vi "SentinelController v35 good v11.vi"() -> ()   [LabVIEW 2011] (continued)
                                n1227 = local read "GPIB Bus 0 traffic"() -> (w1138:string)
                                n1228 = Concatenate Strings(w1138, "\r\n", "Bus 0 waiting on SPOLL" ("string")) -> (w1135:string)
                                n1229 = local write "GPIB Bus 0 traffic"(w1135) -> ()
                                }
                                frame #1 {
                                n1230 = local read "VISA bus 0 resource name out hid"() -> (w1139:refnum<visa-resource-name>)
                                n1231 = local read "VISA bus 0 error out hid"() -> (w1140:errorcluster)
                                n1232 = VISA Discard Events(8:w1140, 11:w1139) -> ()  [unwired: 2 in, 2 out]
                                }
                                frame #2 {
                                n1233 = local read "H1 Ready with sites"() -> (w1143:bool)
                                n1234 = local read "H2 Ready with sites"() -> (w1142:bool)
                                n1235 = Or(x=w1143, y=w1142) -> (x .or. y?=w1141:bool)
                                n1236 = case shown="True" w1141 {
                                frame False {
                                n1237 = flat-sequence {
                                frame #0 {
                                n1238 = Wait (ms)(milliseconds to wait=u32 10) -> ()  [unwired: 1 out]
                                }
                                frame #1 {
                                n1239 = local write "SC handler states hid"(SC_handler_states."waiting on serial poll" ("SC Test Interface States")) -> ()
                                }
                                }
                                }
                                frame True {
                                n1240 = flat-sequence {
                                frame #0 {
                                n1241 = property class="GPIB BoardInterface"(reference=refnum<visa-resource-name> "GPIB0::INTFC", "Device STB"=u8 255 ("Message Based Settings:Device Status Byte")) -> ()  [unwired: 1 in, 2 out]
                                }
                                frame #1 {
                                n1242 = Wait (ms)(milliseconds to wait=u32 5) -> ()  [unwired: 1 out]
                                }
                                frame #2 {
                                n1243 = local read "VISA bus 0 resource name out hid"() -> (w1150:refnum<visa-resource-name>)
                                n1244 = local read "VISA bus 0 error out hid"() -> (w1149:errorcluster)
                                n1245 = local read "GPIB wait timeout hid"() -> (w1158:u32)
                                n1246 = VISA Wait on Event(7:w1158, 8:w1149, 11:w1150) -> (0:w1153:errorcluster, 3:w1152:refnum<visa-resource-name>)  [unwired: 2 in, 2 out]
                                n1247 = local write "VISA bus 0 resource name out hid"(w1152) -> ()
                                n1248 = local write "VISA bus 0 error out hid"(w1153) -> ()
                                n1249 = Unbundle By Name(w1153) -> ("status"=w1155:bool)
                                n1250 = Unbundle By Name(w1153) -> ("code"=w1157:i32)
                                n1251 = Equal?(x=w1157, y=-1073807339) -> (x = y?=w1154:bool)
                                n1252 = Or(x=w1155, y=w1154) -> (x .or. y?=w1151:bool)
                                n1253 = case shown="True" w1151 {
                                tunnel: w1153 -> [_ w1161]
                                tunnel: w1152 -> [_ w1160]
                                frame False {
                                n1254 = local write "SC handler states hid"(SC_handler_states."waiting on event" ("SC Test Interface States")) -> ()
                                }
                                frame True {
                                n1255 = flat-sequence {
                                tunnel: w1161 -> [w1165]
                                tunnel: w1160 -> [w1164]
                                frame #0 {
                                n1256 = VISA Close(VISA resource name=w1164, error in (no error)=w1165) -> (error out=w1163:errorcluster)
                                n1257 = Unbundle By Name(w1163) -> ("status"=w1162:bool)
                                n1258 = local write "VISA bus 0 close error"(w1162) -> ()
                                }
                                frame #1 {
                                n1259 = local write "SC handler states hid"(SC_handler_states."closing bus" ("SC Test Interface States")) -> ()
                                }
                                }
                                }
                                }
                                }
                                }
                                }
                                }
                                }
                                }
                              }
                              frame "reading" {
                                n1260 = local read "VISA bus 0 resource name out hid"() -> (w1175:refnum<visa-resource-name>)
                                n1261 = local read "VISA bus 0 error out hid"() -> (w1174:errorcluster)
                                n1262 = local read "GPIB Bus 0 traffic"() -> (w1177:string)
                                n1263 = VISA Read(VISA resource name=w1175, byte count=256, error in (no error)=w1174) -> (VISA resource name out=w1176:refnum<visa-resource-name>, read buffer=w1167:string, return count=w1170:u32, error out=w1172:errorcluster)
                                n1264 = local write "VISA bus 0 resource name out hid"(w1176) -> ()
                                n1265 = local write "Message from tester hid"(w1167) -> ()
                                n1266 = call <vilib>:"Trim Whitespace.vi"("string"=w1167) -> ("trimmed string"=w1168:string)  [unwired: 1 in]
                                n1267 = Concatenate Strings(w1177, "\r\n", "Bus 0 read: " ("string"), w1168) -> (w1179:string)
                                n1268 = local write "GPIB Bus 0 traffic"(w1179) -> ()
                                n1269 = Greater Than 0?(x=w1170) -> (x > 0?=w1171:bool)
                                n1270 = case shown="True" w1171 {
                                tunnel: w1172 -> [_ w1186]
                                tunnel: w1167 -> [_ w1184]
                                frame False {
                                n1271 = local write "SC handler states hid"(SC_handler_states."waiting on event" ("SC Test Interface States")) -> ()
                                n1272 = Wait (ms)(milliseconds to wait=u32 1) -> ()  [unwired: 1 out]
                                }
                                frame True {
                                n1273 = flat-sequence {
                                tunnel: w1186 -> [w1189]
                                tunnel: [w1188] -> w1185
                                tunnel: w1184 -> [w1188]
                                tunnel: [w1194] -> w1187
                                tunnel: w1185 -> [w1193]
                                tunnel: w1187 -> [w1195]
                                frame #0 {
                                n1274 = local read "Slow for  Diagnostics"() -> (w1191:bool)
                                n1275 = Unbundle By Name(w1189) -> ("status"=w1190:bool)
                                n1276 = local write "GPIB bus 0 read error"(w1190) -> ()
                                n1277 = case shown="True" w1191 {
                                frame False {
                                }
                                frame True {
                                n1278 = local read "GPIB wait time (ms)"() -> (w1192:u32)
                                n1279 = Wait (ms)(milliseconds to wait=w1192) -> ()  [unwired: 1 out]
                                }
                                }
                                }
                                frame #1 {
                                n1280 = call <vilib>:"Trim Whitespace.vi"("string"=w1193) -> ("trimmed string"=w1194:string)  [unwired: 1 in]
                                }
                                frame #2 {
                                n1281 = Match Pattern(string=w1195, regular expression="?") -> (offset past match=w1198:i32)  [unwired: 1 in, 3 out]
                                n1282 = Greater Or Equal To 0?(x=w1198) -> (x >= 0?=w1196:bool)
                                n1283 = case shown="False" w1196 {
                                tunnel: w1195 -> [w1202 w1217]
                                frame False {
                                n1284 = Match Pattern(string=w1202, regular expression=":" ("true string")) -> (offset past match=w1199:i32)  [unwired: 1 in, 3 out]
                                n1285 = Greater Or Equal To 0?(x=w1199) -> (x >= 0?=w1200:bool)
                                n1286 = case shown="False" w1200 {
                                tunnel: w1202 -> [w1205 w1212]
                                frame False {
                                n1287 = call <vilib>:"Space Constant.vi"() -> ("String"=w1206:string)
                                n1288 = Match Pattern(string=w1205, regular expression=w1206) -> (offset past match=w1204:i32)  [unwired: 1 in, 3 out]
                                n1289 = Greater Or Equal To 0?(x=w1204) -> (x >= 0?=w1203:bool)
                                n1290 = case shown="False" w1203 {
                                tunnel: w1205 -> [w1207 w1209]
                                frame False {
                                n1291 = local write "GPIB parsed msg from tester hid"(w1207) -> ()
                                }
                                frame True {
                                n1292 = call <vilib>:"Space Constant.vi"() -> ("String"=w1210:string)
                                n1293 = Match Pattern(string=w1209, regular expression=w1210) -> (before substring=w1208:string)  [unwired: 1 in, 3 out]
                                n1294 = local write "GPIB parsed msg from tester hid"(w1208) -> ()
                                }
                                }
                                }
                                frame True {
                                n1295 = Match Pattern(string=w1212, regular expression=":") -> (before substring=w1211:string)  [unwired: 1 in, 3 out]
                                n1296 = local write "GPIB parsed msg from tester hid"(w1211) -> ()
                                }
                                }
                                }
                                frame True {
                                w1215 = "?" ("regular expression")
                                n1297 = Match Pattern(string=w1217, regular expression=w1215) -> (before substring=w1216:string)  [unwired: 1 in, 3 out]
                                n1298 = Concatenate Strings(w1216, w1215) -> (w1214:string)
                                n1299 = local write "GPIB parsed msg from tester hid"(w1214) -> ()
                                }
                                }
                                }
                                frame #3 {
                                n1300 = local read "GPIB parsed msg from tester hid"() -> (w1218:string)
                                n1301 = case shown="\"BINON\"" w1218 {
                                frame "*IDN?" {
                                n1302 = local write "SC handler states hid"(SC_handler_states."responding to *IDN?" ("SC Test Interface States")) -> ()
                                }
                                frame "SITES?" {
                                n1303 = local read "Tester online"() -> (w1222:bool)
                                n1304 = local read "POWER"() -> (w1220:bool)
                                n1305 = Compound Arithmetic op=AND(w1222, w1220) -> (w1221:bool)
                                n1306 = case shown="True" w1221 {
                                frame False {
                                n1307 = local write "SC handler states hid"(SC_handler_states."closing bus" ("SC virtual handler states")) -> ()
                                }
                                frame True {
                                n1308 = flat-sequence {
                                frame #0 {
                                n1309 = while {
                                stop <- w1225 stop-if-true
                                n1310 = local read "H1 Ready with sites"() -> (w1227:bool)
                                n1311 = local read "H2 Ready with sites"() -> (w1226:bool)
                                n1312 = Or(x=w1227, y=w1226) -> (x .or. y?=w1225:bool)
                                n1313 = Wait (ms)(milliseconds to wait=u32 5) -> ()  [unwired: 1 out]
                                }
                                }
                                frame #1 {
                                n1314 = local write "SC handler states hid"(SC_handler_states."responding to SITES?" ("SC Test Interface States")) -> ()
                                }
                                }
                                }
                                }
                                }
                                frame "Fullsites?" {
                                n1315 = flat-sequence {
                                frame #0 {
                                n1316 = while {
                                stop <- w1230 stop-if-true
                                n1317 = local read "H1 Ready with sites"() -> (w1232:bool)
                                n1318 = local read "H2 Ready with sites"() -> (w1231:bool)
                                n1319 = Or(x=w1232, y=w1231) -> (x .or. y?=w1230:bool)
                                n1320 = Wait (ms)(milliseconds to wait=u32 5) -> ()  [unwired: 1 out]
                                }
                                }
                                frame #1 {
                                n1321 = local write "SC handler states hid"(SC_handler_states."responding to Fullsites?" ("SC Test Interface States")) -> ()
                                }
                                }
                                }
                                frame "HIDN?" {
                                n1322 = local write "SC handler states hid"(SC_handler_states."responding to HIDN?" ("SC Test Interface States")) -> ()
                                }
                                frame "HAND?" {
                                n1323 = local write "SC handler states hid"(SC_handler_states."respond to HAND?" ("SC Test Interface States")) -> ()
                                }
                                frame "A BIN" {
                                n1324 = flat-sequence {
                                frame #0 {
                                n1325 = local read "Message from tester hid"() -> (w1236:string)
                                n1326 = local write "Binning string from tester hid"(w1236) -> ()
                                }
                                frame #1 {
                                n1327 = local write "SC handler states hid"(SC_handler_states."responding to A BIN" ("SC Test Interface States")) -> ()
                                }
                                }
                                }
                                frame "BINON" {
                                n1328 = flat-sequence {
                                frame #0 {
                                # "when this loop unlocks the handlers,\nthe handler interface loops are free to continue\nto send the binning information to their\nrespective handlers."
                                n1329 = local write "H1 Lock"(FALSE ("H1 Lock")) -> ()
                                n1330 = local write "H2 Lock"(FALSE ("H1 Lock")) -> ()
                                n1331 = local read "Message from tester hid"() -> (w1244:string)
                                n1332 = local write "Binning string from tester hid"("") -> ()
                                n1333 = local write "H1 echo hid"("") -> ()
                                n1334 = local write "H2 echo hid"("") -> ()
                                n1335 = local write "Binning string from tester hid"(w1244) -> ()
                                n1336 = local write "Echo state of tester hid"(Echo_tester_states."NO ECHO" ("Echo state of tester hid")) -> ()
                                }
                                frame #1 {
                                n1337 = local write "SC handler states hid"(SC_handler_states."responding to BINON" ("SC Test Interface States")) -> ()
                                }
                                }
                                }
                                frame "ECHOOK" {
                                # "5"
                                n1338 = local write "SC handler states hid"(SC_handler_states."ECHOOK" ("SC Test Interface States")) -> ()
                                n1339 = local write "Echo state of tester hid"(Echo_tester_states."ECHOOK" ("Echo state of tester hid")) -> ()
                                }
                                frame "ECHONG" {
                                n1340 = local write "Echo state of tester hid"(Echo_tester_states."ECHONG" ("Echo state of tester hid")) -> ()
                                n1341 = local write "SC handler states hid"(SC_handler_states."ECHONG" ("SC Test Interface States")) -> ()
                                }
                                frame Default {
                                n1342 = local write "SC handler states hid"(SC_handler_states."responding to unknown command" ("SC Test Interface States")) -> ()
                                }
                                }
                                }
                                }
                                }
                                }
                              }
                              frame "responding to *IDN?" {
                                n1343 = flat-sequence {
                                frame #0 {
                                n1344 = while {
                                stop <- w1256 stop-if-true
                                w1253 = "Sentinel Controller Handler Interface"
                                n1345 = local read "VISA bus 0 resource name out hid"() -> (w1265:refnum<visa-resource-name>)
                                n1346 = local read "VISA bus 0 error out hid"() -> (w1264:errorcluster)
                                n1347 = local read "GPIB Bus 0 traffic"() -> (w1261:string)
                                n1348 = VISA Write(VISA resource name=w1265, write buffer=w1253, error in (no error)=w1264) -> (VISA resource name out=w1263:refnum<visa-resource-name>, return count=w1257:u32, error out=w1262:errorcluster)
                                n1349 = call <vilib>:"Trim Whitespace.vi"("string"=w1253) -> ("trimmed string"=w1254:string)  [unwired: 1 in]
                                n1350 = local write "VISA bus 0 resource name out hid"(w1263) -> ()
                                n1351 = local write "VISA bus 0 error out hid"(w1262) -> ()
                                n1352 = Unbundle By Name(w1262) -> ("status"=w1255:bool)
                                n1353 = Concatenate Strings(w1261, "\r\n", "Bus 0 write: " ("string"), w1254) -> (w1259:string)
                                n1354 = Greater Than 0?(x=w1257) -> (x > 0?=w1256:bool)
                                n1355 = local write "GPIB bus 0 write error"(w1255) -> ()
                                n1356 = local write "GPIB Bus 0 traffic"(w1259) -> ()
                                }
                                }
                                frame #1 {
                                n1357 = local write "SC handler states hid"(SC_handler_states."waiting on event" ("SC Test Interface States")) -> ()
                                }
                                }
                              }
                              frame "respond to HAND?" {
                                n1358 = local read "H1 Lock"() -> (w1269:bool)
                                n1359 = case shown="True" w1269 {
                                frame False {
                                n1360 = local read "H2 Lock"() -> (w1270:bool)
                                n1361 = case shown="True" w1270 {
                                frame False {
                                n1362 = flat-sequence {
                                frame #0 {
                                n1363 = One Button Dialog(message="Fatal error 200:\nThe SC responded to a handler being ready with devices\nto test, but when the SC check for a lock when responding\nto *HAND?, no handler had a lock. \nPlease report this bug to Celerint at www.celerint.com  ") -> ()  [unwired: 1 in, 1 out]
                                }
                                frame #1 {
                                n1364 = local write "SC handler states hid"(SC_handler_states."closing bus" ("SC Test Interface States")) -> ()
                                }
                                }
                                }
                                frame True {
                                n1365 = flat-sequence {
                                frame #0 {
                                n1366 = while {
                                stop <- w1276 stop-if-true
                                w1274 = "H2" ("string")
                                n1367 = local read "VISA bus 0 resource name out hid"() -> (w1282:refnum<visa-resource-name>)
                                n1368 = local read "GPIB Bus 0 traffic"() -> (w1280:string)
                                n1369 = local read "VISA bus 0 error out hid"() -> (w1281:errorcluster)
                                n1370 = call <vilib>:"Trim Whitespace.vi"("string"=w1274) -> ("trimmed string"=w1273:string)  [unwired: 1 in]
                                n1371 = VISA Write(VISA resource name=w1282, write buffer=w1274, error in (no error)=w1281) -> (VISA resource name out=w1283:refnum<visa-resource-name>, return count=w1275:u32, error out=w1284:errorcluster)
                                n1372 = Concatenate Strings(w1280, "\r\n", "H2: Bus 0 write: " ("string"), w1273) -> (w1278:string)
                                n1373 = local write "VISA bus 0 error out hid"(w1284) -> ()
                                n1374 = Unbundle By Name(w1284) -> ("status"=w1285:bool)
                                n1375 = local write "GPIB Bus 0 traffic"(w1278) -> ()
                                n1376 = Greater Than 0?(x=w1275) -> (x > 0?=w1276:bool)
                                n1377 = local write "VISA bus 0 resource name out hid"(w1283) -> ()
                                n1378 = local write "GPIB bus 0 write error"(w1285) -> ()
                                }
                                }
                                frame #1 {
                                n1379 = local write "SC handler states hid"(SC_handler_states."waiting on event" ("SC Test Interface States")) -> ()
                                }
                                }
                                }
                                }
                                }
                                frame True {
                                n1380 = flat-sequence {
                                frame #0 {
                                n1381 = while {
                                stop <- w1290 stop-if-true
                                w1288 = "H1" ("string")
                                n1382 = local read "VISA bus 0 resource name out hid"() -> (w1296:refnum<visa-resource-name>)
                                n1383 = local read "GPIB Bus 0 traffic"() -> (w1294:string)
                                n1384 = local read "VISA bus 0 error out hid"() -> (w1295:errorcluster)
                                n1385 = call <vilib>:"Trim Whitespace.vi"("string"=w1288) -> ("trimmed string"=w1287:string)  [unwired: 1 in]
                                n1386 = Concatenate Strings(w1294, "\r\n", "H1: Bus 0 write: " ("string"), w1287) -> (w1292:string)
                                n1387 = VISA Write(VISA resource name=w1296, write buffer=w1288, error in (no error)=w1295) -> (VISA resource name out=w1297:refnum<visa-resource-name>, return count=w1289:u32, error out=w1298:errorcluster)
                                n1388 = local write "VISA bus 0 resource name out hid"(w1297) -> ()
                                n1389 = local write "VISA bus 0 error out hid"(w1298) -> ()
                                n1390 = Unbundle By Name(w1298) -> ("status"=w1299:bool)
                                n1391 = local write "GPIB Bus 0 traffic"(w1292) -> ()
                                n1392 = Greater Than 0?(x=w1289) -> (x > 0?=w1290:bool)
                                n1393 = local write "GPIB bus 0 write error"(w1299) -> ()
                                }
                                }
                                frame #1 {
                                n1394 = local write "SC handler states hid"(SC_handler_states."waiting on event" ("SC Test Interface States")) -> ()
                                }
                                }
                                }
                                }
                              }
                              frame "responding to HIDN?" {
                                n1395 = local read "H1 Lock"() -> (w1303:bool)
                                n1396 = case shown="True" w1303 {
                                frame False {
                                n1397 = local read "H2 Lock"() -> (w1304:bool)
                                n1398 = case shown="True" w1304 {
                                frame False {
                                n1399 = flat-sequence {
                                frame #0 {
                                n1400 = One Button Dialog(message="Fatal error 201:\nThe SC responded to a handler being ready with devices\nto test, but when the SC check for a lock when responding\nto *HIDN?, no handler had a lock. \nPlease report this bug to Celerint at www.celerint.com  ") -> ()  [unwired: 1 in, 1 out]
                                }
                                frame #1 {
                                n1401 = local write "SC handler states hid"(SC_handler_states."testing" ("SC Test Interface States")) -> ()
                                }
                                }
                                }
                                frame True {
                                n1402 = flat-sequence {
                                frame #0 {
                                n1403 = while {
                                stop <- w1310 stop-if-true
                                n1404 = local read "VISA bus 0 resource name out hid"() -> (w1316:refnum<visa-resource-name>)
                                n1405 = local read "H2 response to *HAND? hid"() -> (w1308:string)
                                n1406 = local read "VISA bus 0 error out hid"() -> (w1315:errorcluster)
                                n1407 = local read "GPIB Bus 0 traffic"() -> (w1314:string)
                                n1408 = VISA Write(VISA resource name=w1316, write buffer=w1308, error in (no error)=w1315) -> (VISA resource name out=w1317:refnum<visa-resource-name>, return count=w1309:u32, error out=w1318:errorcluster)
                                n1409 = call <vilib>:"Trim Whitespace.vi"("string"=w1308) -> ("trimmed string"=w1307:string)  [unwired: 1 in]
                                n1410 = local write "VISA bus 0 error out hid"(w1318) -> ()
                                n1411 = Unbundle By Name(w1318) -> ("status"=w1319:bool)
                                n1412 = Concatenate Strings(w1314, "\r\n", "H2: Bus 0 write: " ("string"), w1307) -> (w1312:string)
                                n1413 = Greater Than 0?(x=w1309) -> (x > 0?=w1310:bool)
                                n1414 = local write "VISA bus 0 resource name out hid"(w1317) -> ()
                                n1415 = local write "GPIB Bus 0 traffic"(w1312) -> ()
                                n1416 = local write "GPIB bus 0 write error"(w1319) -> ()
                                }
                                }
                                frame #1 {
                                n1417 = local write "SC handler states hid"(SC_handler_states."waiting on event" ("SC Test Interface States")) -> ()
                                }
                                }
                                }
                                }
                                }
                                frame True {
                                n1418 = flat-sequence {
                                frame #0 {
                                n1419 = while {
                                stop <- w1324 stop-if-true
                                n1420 = local read "VISA bus 0 resource name out hid"() -> (w1330:refnum<visa-resource-name>)
                                n1421 = local read "H1 response to *HAND? hid"() -> (w1322:string)
                                n1422 = local read "VISA bus 0 error out hid"() -> (w1329:errorcluster)
                                n1423 = local read "GPIB Bus 0 traffic"() -> (w1328:string)
                                n1424 = call <vilib>:"Trim Whitespace.vi"("string"=w1322) -> ("trimmed string"=w1321:string)  [unwired: 1 in]
                                n1425 = VISA Write(VISA resource name=w1330, write buffer=w1322, error in (no error)=w1329) -> (VISA resource name out=w1331:refnum<visa-resource-name>, return count=w1323:u32, error out=w1332:errorcluster)
                                n1426 = local write "VISA bus 0 resource name out hid"(w1331) -> ()
                                n1427 = local write "VISA bus 0 error out hid"(w1332) -> ()
                                n1428 = Unbundle By Name(w1332) -> ("status"=w1333:bool)
                                n1429 = Concatenate Strings(w1328, "\r\n", "H1: Bus 0 write: " ("string"), w1321) -> (w1326:string)
                                n1430 = Greater Than 0?(x=w1323) -> (x > 0?=w1324:bool)
                                n1431 = local write "GPIB Bus 0 traffic"(w1326) -> ()
                                n1432 = local write "GPIB bus 0 write error"(w1333) -> ()
                                }
                                }
                                frame #1 {
                                n1433 = local write "SC handler states hid"(SC_handler_states."waiting on event" ("SC Test Interface States")) -> ()
                                }
                                }
                                }
                                }
                              }
                              frame "responding to Fullsites?" {
                                n1434 = flat-sequence {
                                frame #0 {
                                n1435 = local read "Last locked handler hid"() -> (w1337:enum16{"H1", "H2"})
                                n1436 = case shown="\"H2\"" w1337 {
                                frame "H1", Default {
                                n1437 = local read "H2 Ready with sites"() -> (w1338:bool)
                                n1438 = case shown="True" w1338 {
                                frame False {
                                n1439 = local read "H1 Ready with sites"() -> (w1339:bool)
                                n1440 = case shown="True" w1339 {
                                frame False {
                                # "end up here only if neither handler is waiting and ready"
                                n1441 = One Button Dialog(message="Ouch", button name ("OK")="crash") -> ()  [unwired: 1 out]
                                }
                                frame True {
                                n1442 = flat-sequence {
                                frame #0 {
                                n1443 = while {
                                stop <- w1344 stop-if-true
                                n1444 = local read "VISA bus 0 resource name out hid"() -> (w1352:refnum<visa-resource-name>)
                                n1445 = local read "H1 FULLSITES? response hid"() -> (w1343:string)
                                n1446 = local read "VISA bus 0 error out hid"() -> (w1353:errorcluster)
                                n1447 = VISA Write(VISA resource name=w1352, write buffer=w1343, error in (no error)=w1353) -> (VISA resource name out=w1351:refnum<visa-resource-name>, return count=w1345:u32, error out=w1350:errorcluster)
                                n1448 = local write "VISA bus 0 resource name out hid"(w1351) -> ()
                                n1449 = Unbundle By Name(w1350) -> ("status"=w1354:bool)
                                n1450 = local write "VISA bus 0 error out hid"(w1350) -> ()
                                n1451 = Greater Than 0?(x=w1345) -> (x > 0?=w1344:bool)
                                n1452 = call <vilib>:"Trim Whitespace.vi"("string"=w1343) -> ("trimmed string"=w1342:string)  [unwired: 1 in]
                                n1453 = local write "GPIB bus 0 write error"(w1354) -> ()
                                n1454 = Concatenate Strings("H1: Tester test cycle start" ("string"), "\r\n", "Bus 0 write: " ("string"), w1342) -> (w1348:string)
                                n1455 = local write "GPIB Bus 0 traffic"(w1348) -> ()
                                }
                                }
                                frame #1 {
                                n1456 = local read "H1 loop counter hid"() -> (w1358:u32)
                                n1457 = local write "Last locked handler hid"(enum16{"H1", "H2"}."H1" ("Last locked handler hid")) -> ()
                                n1458 = Increment(x=w1358) -> (x+1=w1357:u32)
                                n1459 = local write "H1 Lock"(TRUE ("H1 Lock")) -> ()
                                n1460 = local write "H1 loop counter hid"(w1357) -> ()
                                }
                                }
                                }
                                }
                                }
                                frame True {
                                n1461 = flat-sequence {
                                frame #0 {
                                n1462 = while {
                                stop <- w1362 stop-if-true
                                n1463 = local read "VISA bus 0 resource name out hid"() -> (w1369:refnum<visa-resource-name>)
                                n1464 = local read "H2 FULLSITES? response hid"() -> (w1360:string)
                                n1465 = local read "VISA bus 0 error out hid"() -> (w1370:errorcluster)
                                n1466 = VISA Write(VISA resource name=w1369, write buffer=w1360, error in (no error)=w1370) -> (VISA resource name out=w1368:refnum<visa-resource-name>, return count=w1361:u32, error out=w1367:errorcluster)
                                n1467 = local write "VISA bus 0 resource name out hid"(w1368) -> ()
                                n1468 = Unbundle By Name(w1367) -> ("status"=w1371:bool)
                                n1469 = local write "VISA bus 0 error out hid"(w1367) -> ()
                                n1470 = Greater Than 0?(x=w1361) -> (x > 0?=w1362:bool)
                                n1471 = call <vilib>:"Trim Whitespace.vi"("string"=w1360) -> ("trimmed string"=w1359:string)  [unwired: 1 in]
                                n1472 = local write "GPIB bus 0 write error"(w1371) -> ()
                                n1473 = Concatenate Strings("H2: Tester test cycle start" ("string"), "\r\n", "Bus 0 write: " ("string"), w1359) -> (w1365:string)
                                n1474 = local write "GPIB Bus 0 traffic"(w1365) -> ()
                                }
                                }
                                frame #1 {
                                n1475 = local read "H2 loop counter hid"() -> (w1374:u32)
                                n1476 = local write "Last locked handler hid"(enum16{"H1", "H2"}."H2" ("Last locked handler hid")) -> ()
                                n1477 = local write "H2 Lock"(TRUE ("H2 Lock")) -> ()
                                n1478 = Increment(x=w1374) -> (x+1=w1375:u32)
                                n1479 = local write "H2 loop counter hid"(w1375) -> ()
                                }
                                }
                                }
                                }
                                }
                                frame "H2" {
                                n1480 = local read "H1 Ready with sites"() -> (w1376:bool)
                                n1481 = case shown="True" w1376 {
                                frame False {
                                n1482 = local read "H2 Ready with sites"() -> (w1377:bool)
                                n1483 = case shown="True" w1377 {
                                frame False {
                                # "end up here only if neither handler is waiting and ready"
                                }
                                frame True {
                                n1484 = flat-sequence {
                                frame #0 {
                                n1485 = while {
                                stop <- w1381 stop-if-true
                                n1486 = local read "VISA bus 0 resource name out hid"() -> (w1388:refnum<visa-resource-name>)
                                n1487 = local read "H2 FULLSITES? response hid"() -> (w1378:string)
                                n1488 = local read "VISA bus 0 error out hid"() -> (w1389:errorcluster)
                                n1489 = VISA Write(VISA resource name=w1388, write buffer=w1378, error in (no error)=w1389) -> (VISA resource name out=w1387:refnum<visa-resource-name>, return count=w1380:u32, error out=w1386:errorcluster)
                                n1490 = local write "VISA bus 0 resource name out hid"(w1387) -> ()
                                n1491 = Unbundle By Name(w1386) -> ("status"=w1390:bool)
                                n1492 = local write "VISA bus 0 error out hid"(w1386) -> ()
                                n1493 = call <vilib>:"Trim Whitespace.vi"("string"=w1378) -> ("trimmed string"=w1379:string)  [unwired: 1 in]
                                n1494 = Greater Than 0?(x=w1380) -> (x > 0?=w1381:bool)
                                n1495 = Concatenate Strings("H2: Tester test cycle start" ("string"), "\r\n", "Bus 0 write: " ("string"), w1379) -> (w1384:string)
                                n1496 = local write "GPIB bus 0 write error"(w1390) -> ()
                                n1497 = local write "GPIB Bus 0 traffic"(w1384) -> ()
                                }
                                }
                                frame #1 {
                                n1498 = local read "H2 loop counter hid"() -> (w1393:u32)
                                n1499 = local write "H2 Lock"(TRUE ("H2 Lock")) -> ()
                                n1500 = local write "Last locked handler hid"(enum16{"H1", "H2"}."H2" ("Last locked handler hid")) -> ()
                                n1501 = Increment(x=w1393) -> (x+1=w1394:u32)
                                n1502 = local write "H2 loop counter hid"(w1394) -> ()
                                }
                                }
                                }
                                }
                                }
                                frame True {
                                n1503 = flat-sequence {
                                frame #0 {
                                n1504 = while {
                                stop <- w1397 stop-if-true
                                n1505 = local read "VISA bus 0 resource name out hid"() -> (w1405:refnum<visa-resource-name>)
                                n1506 = local read "H1 FULLSITES? response hid"() -> (w1395:string)
                                n1507 = local read "VISA bus 0 error out hid"() -> (w1406:errorcluster)
                                n1508 = VISA Write(VISA resource name=w1405, write buffer=w1395, error in (no error)=w1406) -> (VISA resource name out=w1404:refnum<visa-resource-name>, return count=w1398:u32, error out=w1403:errorcluster)
                                n1509 = local write "VISA bus 0 resource name out hid"(w1404) -> ()
                                n1510 = Unbundle By Name(w1403) -> ("status"=w1407:bool)
                                n1511 = local write "VISA bus 0 error out hid"(w1403) -> ()
                                n1512 = Greater Than 0?(x=w1398) -> (x > 0?=w1397:bool)
                                n1513 = call <vilib>:"Trim Whitespace.vi"("string"=w1395) -> ("trimmed string"=w1396:string)  [unwired: 1 in]
                                n1514 = local write "GPIB bus 0 write error"(w1407) -> ()
                                n1515 = Concatenate Strings("H1: Tester test cycle start" ("string"), "\r\n", "Bus 0 write: " ("string"), w1396) -> (w1401:string)
                                n1516 = local write "GPIB Bus 0 traffic"(w1401) -> ()
                                }
                                }
                                frame #1 {
                                n1517 = local read "H1 loop counter hid"() -> (w1411:u32)
                                n1518 = local write "Last locked handler hid"(enum16{"H1", "H2"}."H1" ("Last locked handler hid")) -> ()
                                n1519 = local write "H1 Lock"(TRUE ("H1 Lock")) -> ()
                                n1520 = Increment(x=w1411) -> (x+1=w1410:u32)
                                n1521 = local write "H1 loop counter hid"(w1410) -> ()
                                }
                                }
                                }
                                }
                                }
                                }
                                }
                                frame #1 {
                                n1522 = local write "SC handler states hid"(SC_handler_states."testing" ("SC Test Interface States")) -> ()
                                }
                                }
                              }
                              frame "testing" {
                                n1523 = flat-sequence {
                                tunnel: w1423 -> [w1427]
                                tunnel: w1424 -> [w1428]
                                tunnel: [w1426] -> w1420
                                tunnel: [w1425] -> w1419
                                tunnel: w1420 -> [w1444]
                                tunnel: [w1444] -> w1418
                                tunnel: w1419 -> [w1443]
                                tunnel: [w1443] -> w1417
                                tunnel: w1418 -> [w1446]
                                tunnel: w1417 -> [w1445]
                                tunnel: [w1446] -> w1416
                                tunnel: [w1445] -> w1415
                                tunnel: w1416 -> [w1455]
                                tunnel: w1415 -> [w1454]
                                tunnel: [w1455] -> w1414
                                tunnel: [w1454] -> w1413
                                tunnel: [w1457] -> w1422
                                tunnel: [w1458] -> w1421
                                tunnel: w1414 -> [w1458]
                                tunnel: w1413 -> [w1457]
                                frame #0 {
                                n1524 = local read "SC measured test time hid"() -> (w1429:dbl)
                                n1525 = local read "SC measured wait time hid"() -> (w1430:dbl)
                                n1526 = local read "Tester loop counter hid"() -> (w1432:u32)
                                n1527 = Add(x=w1429, y=w1430) -> (x+y=w1436:dbl)
                                n1528 = local read "Utilization averaging"() -> (w1431:i32)
                                n1529 = Divide(x=w1429, y=w1436) -> (x/y=w1437:dbl)
                                n1530 = Multiply(x=100.0, y=w1437) -> (x*y=w1433:dbl)
                                n1531 = call "moving_avg_core.vi"("Array in"=w1427, "avg"=w1431, "accumulator in"=w1428, "i"=w1432, "data in"=w1433) -> ("Array out"=w1426:dbl[], "accumulator out"=w1425:dbl, "rolling avg out"=w1434:dbl)  [unwired: 4 in]
                                n1532 = Bundle(w1433, "rolling avg out"=w1434) -> (w1435:cluster{dbl, "rolling avg out":dbl})  [unwired: 1 in]
                                n1533 = local write "Sys utilization"(w1434) -> ()
                                n1534 = local write "SysUtilMon"(w1435) -> ()
                                }
                                frame #1 {
                                # "empty binning string wiill hold handlers at BINON until valid"
                                n1535 = local read "H1 loop counter hid"() -> (w1441:u32)
                                n1536 = Increment(x=w1441) -> (x+1=w1442:u32)
                                n1537 = property class="GPIB BoardInterface"(reference=refnum<visa-resource-name> "GPIB0::INTFC", "Device STB"=u8 0 ("Message Based Settings:Device Status Byte")) -> ()  [unwired: 1 in, 2 out]
                                n1538 = local write "H1 loop counter hid"(w1442) -> ()
                                }
                                frame #2 {
                                n1539 = Tick Count (ms)() -> (millisecond timer value=w1448:u32)
                                n1540 = Tick Count (ms)() -> (millisecond timer value=w1447:u32)
                                n1541 = local write "tester wt end hid"(w1448) -> ()
                                n1542 = local write "tester tt start hid"(w1447) -> ()
                                }
                                frame #3 {
                                n1543 = local read "tester wt start hid"() -> (w1452:u32)
                                n1544 = local read "tester wt end hid"() -> (w1453:u32)
                                n1545 = Subtract(x=w1453, y=w1452) -> (x-y=w1451:u32)
                                n1546 = Divide(x=w1451, y=u32 1000) -> (x/y=w1449:dbl)
                                n1547 = local write "SC measured wait time hid"(w1449) -> ()
                                }
                                frame #4 {
                                n1548 = local write "SC handler states hid"(SC_handler_states."waiting on event" ("SC Test Interface States")) -> ()
                                }
                                }
                              }
                              frame "responding to SITES?" {
                                n1549 = flat-sequence {
                                frame #0 {
                                # "This is the engine that decides if H1 is checked first or H2"
                                n1550 = local read "Last locked handler hid"() -> (w1461:enum16{"H1", "H2"})
                                n1551 = case shown="\"H2\"" w1461 {
                                frame "H1", Default {
                                n1552 = local read "H2 Ready with sites"() -> (w1462:bool)
                                n1553 = case shown="True" w1462 {
                                frame False {
                                n1554 = local read "H1 Ready with sites"() -> (w1463:bool)
                                n1555 = case shown="True" w1463 {
                                frame False {
                                # "end up here only if neither handler is waiting and ready"
                                }
                                frame True {
                                n1556 = flat-sequence {
                                frame #0 {
                                n1557 = local write "H2 Lock"(FALSE ("H1 Lock")) -> ()
                                n1558 = local write "H1 Lock"(TRUE ("H1 Lock")) -> ()
                                n1559 = local write "Last locked handler hid"(enum16{"H1", "H2"}."H1" ("Last locked handler")) -> ()
                                }
                                frame #1 {
                                n1560 = while {
                                stop <- w1469 stop-if-true
                                n1561 = local read "VISA bus 0 resource name out hid"() -> (w1477:refnum<visa-resource-name>)
                                n1562 = local read "VISA bus 0 error out hid"() -> (w1478:errorcluster)
                                n1563 = local read "H1 SITES? response hid"() -> (w1467:string)
                                n1564 = VISA Write(VISA resource name=w1477, write buffer=w1467, error in (no error)=w1478) -> (VISA resource name out=w1476:refnum<visa-resource-name>, return count=w1470:u32, error out=w1475:errorcluster)
                                n1565 = local write "VISA bus 0 resource name out hid"(w1476) -> ()
                                n1566 = Unbundle By Name(w1475) -> ("status"=w1479:bool)
                                n1567 = local write "VISA bus 0 error out hid"(w1475) -> ()
                                n1568 = call <vilib>:"Trim Whitespace.vi"("string"=w1467) -> ("trimmed string"=w1468:string)  [unwired: 1 in]
                                n1569 = Greater Than 0?(x=w1470) -> (x > 0?=w1469:bool)
                                n1570 = Concatenate Strings("H1: Tester test cycle start" ("string"), "\r\n", "Bus 0 write: " ("string"), w1468) -> (w1473:string)
                                n1571 = local write "GPIB bus 0 write error"(w1479) -> ()
                                n1572 = local write "GPIB Bus 0 traffic"(w1473) -> ()
                                }
                                }
                                }
                                }
                                }
                                }
                                frame True {
                                n1573 = flat-sequence {
                                frame #0 {
                                n1574 = local write "H1 Lock"(FALSE ("H1 Lock")) -> ()
                                n1575 = local write "H2 Lock"(TRUE ("H1 Lock")) -> ()
                                n1576 = local write "Last locked handler hid"(enum16{"H1", "H2"}."H2" ("Last locked handler")) -> ()
                                }
                                frame #1 {
                                n1577 = while {
                                stop <- w1486 stop-if-true
                                n1578 = local read "VISA bus 0 resource name out hid"() -> (w1493:refnum<visa-resource-name>)
                                n1579 = local read "VISA bus 0 error out hid"() -> (w1494:errorcluster)
                                n1580 = local read "H2 SITES? response hid"() -> (w1483:string)
                                n1581 = VISA Write(VISA resource name=w1493, write buffer=w1483, error in (no error)=w1494) -> (VISA resource name out=w1492:refnum<visa-resource-name>, return count=w1485:u32, error out=w1491:errorcluster)
                                n1582 = local write "VISA bus 0 resource name out hid"(w1492) -> ()
                                n1583 = Unbundle By Name(w1491) -> ("status"=w1495:bool)
                                n1584 = local write "VISA bus 0 error out hid"(w1491) -> ()
                                n1585 = Greater Than 0?(x=w1485) -> (x > 0?=w1486:bool)
                                n1586 = call <vilib>:"Trim Whitespace.vi"("string"=w1483) -> ("trimmed string"=w1484:string)  [unwired: 1 in]
                                n1587 = local write "GPIB bus 0 write error"(w1495) -> ()
                                n1588 = Concatenate Strings("H2: Tester test cycle start" ("string"), "\r\n", "Bus 0 write: " ("string"), w1484) -> (w1489:string)
                                n1589 = local write "GPIB Bus 0 traffic"(w1489) -> ()
                                }
                                }
                                frame #2 {
                                n1590 = local read "H2 loop counter hid"() -> (w1496:u32)
                                n1591 = Increment(x=w1496) -> (x+1=w1497:u32)
                                n1592 = local write "H2 loop counter hid"(w1497) -> ()
                                }
                                }
                                }
                                }
                                }
                                frame "H2" {
                                n1593 = local read "H1 Ready with sites"() -> (w1498:bool)
                                n1594 = case shown="True" w1498 {
                                frame False {
                                n1595 = local read "H2 Ready with sites"() -> (w1499:bool)
                                n1596 = case shown="True" w1499 {
                                frame False {
                                # "end up here only if neither handler is waiting and ready"
                                }
                                frame True {
                                n1597 = flat-sequence {
                                frame #0 {
                                n1598 = local write "H2 Lock"(TRUE ("H1 Lock")) -> ()
                                n1599 = local write "H1 Lock"(FALSE ("H1 Lock")) -> ()
                                n1600 = local write "Last locked handler hid"(enum16{"H1", "H2"}."H2" ("Last locked handler")) -> ()
                                }
                                frame #1 {
                                n1601 = while {
                                stop <- w1506 stop-if-true
                                n1602 = local read "VISA bus 0 resource name out hid"() -> (w1513:refnum<visa-resource-name>)
                                n1603 = local read "VISA bus 0 error out hid"() -> (w1514:errorcluster)
                                n1604 = local read "H2 SITES? response hid"() -> (w1503:string)
                                n1605 = VISA Write(VISA resource name=w1513, write buffer=w1503, error in (no error)=w1514) -> (VISA resource name out=w1512:refnum<visa-resource-name>, return count=w1505:u32, error out=w1511:errorcluster)
                                n1606 = local write "VISA bus 0 resource name out hid"(w1512) -> ()
                                n1607 = Unbundle By Name(w1511) -> ("status"=w1515:bool)
                                n1608 = local write "VISA bus 0 error out hid"(w1511) -> ()
                                n1609 = Greater Than 0?(x=w1505) -> (x > 0?=w1506:bool)
                                n1610 = call <vilib>:"Trim Whitespace.vi"("string"=w1503) -> ("trimmed string"=w1504:string)  [unwired: 1 in]
                                n1611 = Concatenate Strings("H2: Tester test cycle start" ("string"), "\r\n", "Bus 0 write: " ("string"), w1504) -> (w1509:string)
                                n1612 = local write "GPIB bus 0 write error"(w1515) -> ()
                                n1613 = local write "GPIB Bus 0 traffic"(w1509) -> ()
                                }
                                }
                                frame #2 {
                                n1614 = local read "H2 loop counter hid"() -> (w1516:u32)
                                n1615 = Increment(x=w1516) -> (x+1=w1517:u32)
                                n1616 = local write "H2 loop counter hid"(w1517) -> ()
                                }
                                }
                                }
                                }
                                }
                                frame True {
                                n1617 = flat-sequence {
                                frame #0 {
                                n1618 = local write "Last locked handler hid"(enum16{"H1", "H2"}."H1" ("Last locked handler")) -> ()
                                }
                                frame #1 {
                                n1619 = while {
                                stop <- w1521 stop-if-true
                                n1620 = local read "VISA bus 0 resource name out hid"() -> (w1529:refnum<visa-resource-name>)
                                n1621 = local read "VISA bus 0 error out hid"() -> (w1530:errorcluster)
                                n1622 = local read "H1 SITES? response hid"() -> (w1519:string)
                                n1623 = VISA Write(VISA resource name=w1529, write buffer=w1519, error in (no error)=w1530) -> (VISA resource name out=w1528:refnum<visa-resource-name>, return count=w1522:u32, error out=w1527:errorcluster)
                                n1624 = local write "VISA bus 0 resource name out hid"(w1528) -> ()
                                n1625 = Unbundle By Name(w1527) -> ("status"=w1531:bool)
                                n1626 = local write "VISA bus 0 error out hid"(w1527) -> ()
                                n1627 = Greater Than 0?(x=w1522) -> (x > 0?=w1521:bool)
                                n1628 = call <vilib>:"Trim Whitespace.vi"("string"=w1519) -> ("trimmed string"=w1520:string)  [unwired: 1 in]
                                n1629 = local write "GPIB bus 0 write error"(w1531) -> ()
                                n1630 = Concatenate Strings("H1: Tester test cycle start" ("string"), "\r\n", "Bus 0 write: " ("string"), w1520) -> (w1525:string)
                                n1631 = local write "GPIB Bus 0 traffic"(w1525) -> ()
                                }
                                }
                                frame #2 {
                                n1632 = local read "H1 loop counter hid"() -> (w1533:u32)
                                n1633 = Increment(x=w1533) -> (x+1=w1532:u32)
                                n1634 = local write "H1 loop counter hid"(w1532) -> ()
                                }
                                }
                                }
                                }
                                }
                                }
                                }
                                frame #1 {
                                n1635 = local write "SC handler states hid"(SC_handler_states."testing" ("SC Test Interface States")) -> ()
                                }
                                }
                              }
                              frame "responding to A BIN" {
                                n1636 = flat-sequence {
                                frame #0 {
                                n1637 = local read "H1 Lock"() -> (w1537:bool)
                                n1638 = case shown="True" w1537 {
                                frame False {
                                n1639 = local read "H2 Lock"() -> (w1538:bool)
                                n1640 = case shown="True" w1538 {
                                frame False {
                                }
                                frame True {
                                n1641 = local read "GPIB Bus 0 traffic"() -> (w1542:string)
                                n1642 = Concatenate Strings(w1542, "\r\n", "Bus 0: binning" ("string")) -> (w1540:string)
                                n1643 = local write "GPIB Bus 0 traffic"(w1540) -> ()
                                }
                                }
                                }
                                frame True {
                                n1644 = local read "GPIB Bus 0 traffic"() -> (w1546:string)
                                n1645 = Concatenate Strings(w1546, "\r\n", "Bus 0: binning" ("string")) -> (w1544:string)
                                n1646 = local write "GPIB Bus 0 traffic"(w1544) -> ()
                                }
                                }
                                }
                                frame #1 {
                                n1647 = Tick Count (ms)() -> (millisecond timer value=w1548:u32)
                                n1648 = Tick Count (ms)() -> (millisecond timer value=w1547:u32)
                                n1649 = local write "tester tt end hid"(w1548) -> ()
                                n1650 = local write "tester wt start hid"(w1547) -> ()
                                }
                                frame #2 {
